vi "Waveform Example.vi"() -> ()   [LabVIEW 2016]
uses:
  controls/Microscope Settings.ctl
  controls/CameraState.ctl
  controls/ModeEnum.ctl
  <vilib>/DAQmx/write.llb/DAQmx Write (Digital 1D Wfm NChan NSamp).vi
  <vilib>/DAQmx/write.llb/DAQmx Write (Analog 1D Wfm NChan NSamp).vi
  <vilib>/Waveform/WDTOps.llb/WDT Number of Waveform Samples DBL.vi
  <vilib>/DAQmx/configure/timing.llb/DAQmx Timing (Sample Clock).vi
  <vilib>/Waveform/DWDTOps.llb/DWDT Uncompress Digital.vi
  <vilib>/DAQmx/miscellaneous.llb/DAQmx Fill In Error Info.vi
  <vilib>/Waveform/WDTOps.llb/WDT Waveform Duration DBL.vi
  <vilib>/DAQmx/create/channels.llb/DAQmx Create Channel (AO-Voltage-Basic).vi
  <vilib>/DAQmx/create/channels.llb/DAQmx Create Channel (DO-Digital Output).vi
  controls/PinOut.ctl
  controls/PinOut2.ctl
panel:
  out "Numeric 3":i32
  out "Numeric 2":i32
  in  "Tab Control":enum32{"Camera Settings", "Recording"}(tab)
  out "error IO":errorcluster
  out "Duration":string
  in  "Microscope Settings":T1={"Mode"=enum."XY", "Slit"={"Scanning Mode"=12.0, "Slit Width /%"=5.0}, "Colour"=[{"Laser"=enum."561", "Filter"=4}], "Exposure/ms"=40.0, "Piezo Position /um"=0.0, "ROI"={"X"={"Start /px"=0.0, "Step /px"=1.0, "Range /px"=2048.0}, "Y"={"Start /px"=0.0, "Step /px"=1.0, "Range /px"=2048.0}, "Z "={"Start /um"=0.0, "Step/um"=1.0, "Range /um"=100.0}, "T "={"Start /s"=0.0, "Step /s"=1.0, "Range /s"=100.0}}, "Samples per millisecond"=100.0, "Relax/ms"=10.0, "Readout Direction"=2.0, "Trigger Source"=2.0, "Camera Delay /ms"=11.0, "Under Scan /ms"=5.0, "Calibration Coordinates"={"Top Left"=[-4.418670520231216, -0.1592138728323702, 10.0], "Top Right"=[-9.501965317919073, -0.1592138728323702, 10.0], "Bottom Left"=[-4.4508670520231215, 0.0, 0.0], "Bottom Right"=[-9.53757225433526, 0.0, 0.0], "Waveforms"={"Analogue Out"=[], "Digital Out"=[]}}} {"Under Scan /ms" min=0.0 max=10.0 step=0.05; "ROI"."T"."Range /s" min=0.0 max=10.0 step=0.05 format="%<%H:%M:%S>t"; "ROI"."T"."Step /s" min=0.0 max=10.0 step=0.05 format="%<%M:%S%2u>t"; "ROI"."T"."Start /s" min=0.0 max=10.0 step=0.05 format="%<%M:%S%2u>t"; "ROI"."X"."Range /px" min=0.0 max=10.0 step=0.05; "ROI"."X"."Step /px" min=0.0 max=10.0 step=0.05; "ROI"."X"."Start /px" min=0.0 max=10.0 step=0.05; "ROI"."Y"."Range /px" min=0.0 max=10.0 step=0.05; "ROI"."Y"."Step /px" min=0.0 max=10.0 step=0.05; "ROI"."Y"."Start /px" min=0.0 max=10.0 step=0.05; "ROI"."Z"."Range /um" min=0.0 max=10.0 step=0.05; "ROI"."Z"."Step/um" min=0.0001 max=10.0 step=0.05; "ROI"."Z"."Start /um" min=0.0 max=10.0 step=0.05; "Colour"."Filter" items=["Empty"=1, ""=2, ""=3, "561"=4, ""=5, "488"=6]; "Camera Delay /ms" min=0.0 max=10.0 step=0.05; "Trigger Source" items=["Internal"=1.0, "External"=2.0]; "Readout Direction" items=["Forward"=1.0, "Backward"=2.0]; "Slit"."Scanning Mode" items=["Full Frame"=1.0, "Slit Scanning"=12.0]; "Piezo Position /um" min=0.0 max=10.0 step=0.05}
  out "Mixed Signal Graph 2":cluster{waveform(dbl)[], digitalwaveform[]}(graph)
  in  "stop":bool
  in  "Signals Debugger":bool
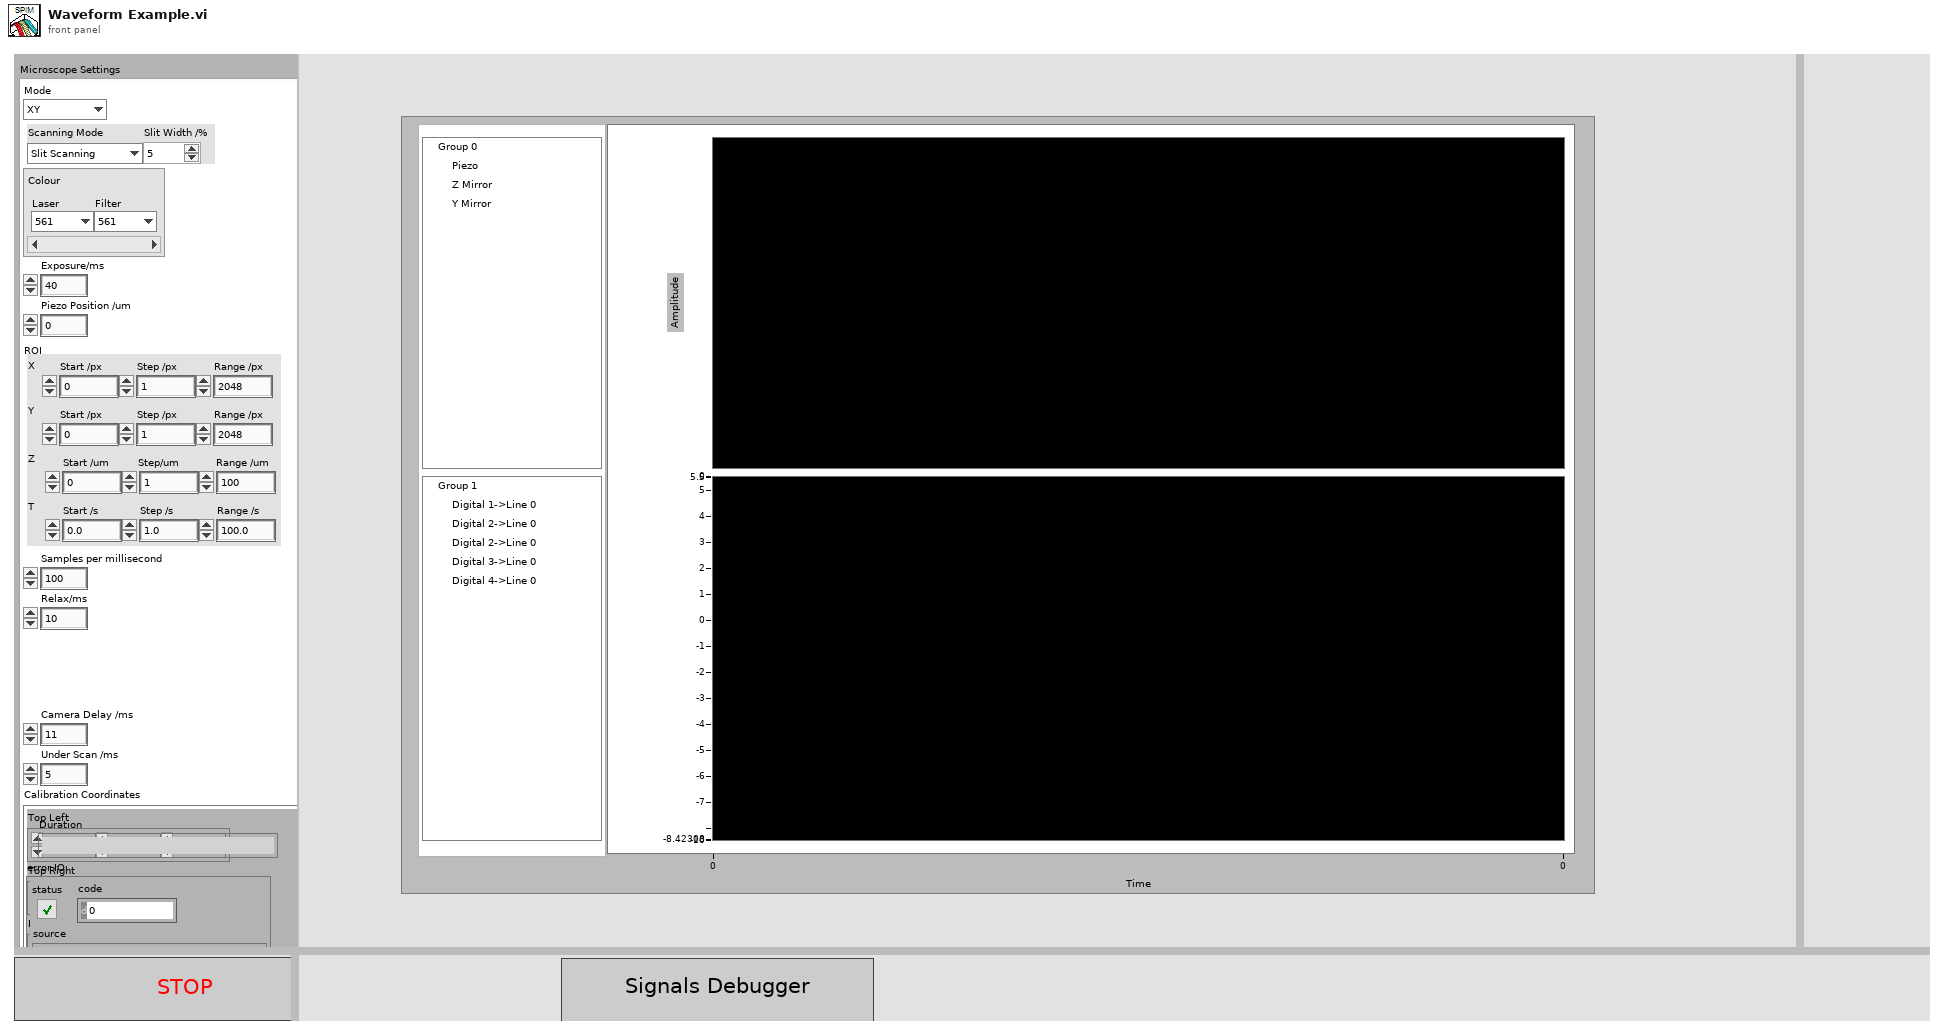
[diagram p1: front panel]
types:
  T1 = typedef "Microscope Settings.ctl" = cluster{"Mode":enum16{"Brightfield", "X", "XY", "XYZ", "XYZT", "XYZC", "Tweezers", "Virus"}, "Slit":cluster{"Scanning Mode":dbl, "Slit Width /%":dbl}, "Colour":cluster{"Laser":enum16{"Brightfield", "445", "488", "561", "647"}, "Filter":u16}[], "Exposure/ms":dbl, "Piezo Position /um":dbl, "ROI":cluster{"X":cluster{"Start /px":dbl, "Step /px":dbl, "Range /px":dbl}, "Y":cluster{"Start /px":dbl, "Step /px":dbl, "Range /px":dbl}, "Z ":cluster{"Start /um":dbl, "Step/um":dbl, "Range /um":dbl}, "T ":cluster{"Start /s":dbl, "Step /s":dbl, "Range /s":dbl}}, "Samples per millisecond":dbl, "Relax/ms":dbl, "Readout Direction":dbl, "Trigger Source":dbl, "Camera Delay /ms":dbl, "Under Scan /ms":dbl, "Calibration Coordinates":cluster{"Top Left":dbl[], "Top Right":dbl[], "Bottom Left":dbl[], "Bottom Right":dbl[], "Waveforms":cluster{"Analogue Out":waveform(dbl)[], "Digital Out":digitalwaveform[]}}}
  T2 = typedef "CameraState.ctl" = enum16{"init", "active", "deinit"}
  T3 = typedef "ModeEnum.ctl" = enum16{"Idle", "Init", "generateWaves", "runWaves", "runWavesCont", "endWavesCont", "stop"}
  T4 = enum16{"Stop", "Idle", "Update", "Run Waves", ""}
  T5 = typedef "PinOut.ctl" = string
  T6 = enum32{"Invalid", "Standard", "Closed", "Hidden", "Minimized", "Maximized"}
  T7 = cluster{"Analogue Out":waveform(dbl)[], "Digital Out":digitalwaveform[]}
  T8 = cluster{enum16{"Stop", "Idle", "Update", "Run Waves", ""}, "Microscope Settings":T1}
  T9 = typedef "PinOut2.ctl" = string
  T10 = enum16{"Brightfield", "X", "XY", "XYZ", "XYZT", "XYZC", "Tweezers", "Virus"}
  T11 = cluster{"Start /um":dbl, "Step/um":dbl, "Range /um":dbl}
  T12 = cluster{"Analogue Out out":waveform(dbl)[], "Digital Out out":digitalwaveform[]}
  T13 = cluster{"Start /s":dbl, "Step /s":dbl, "Range /s":dbl}
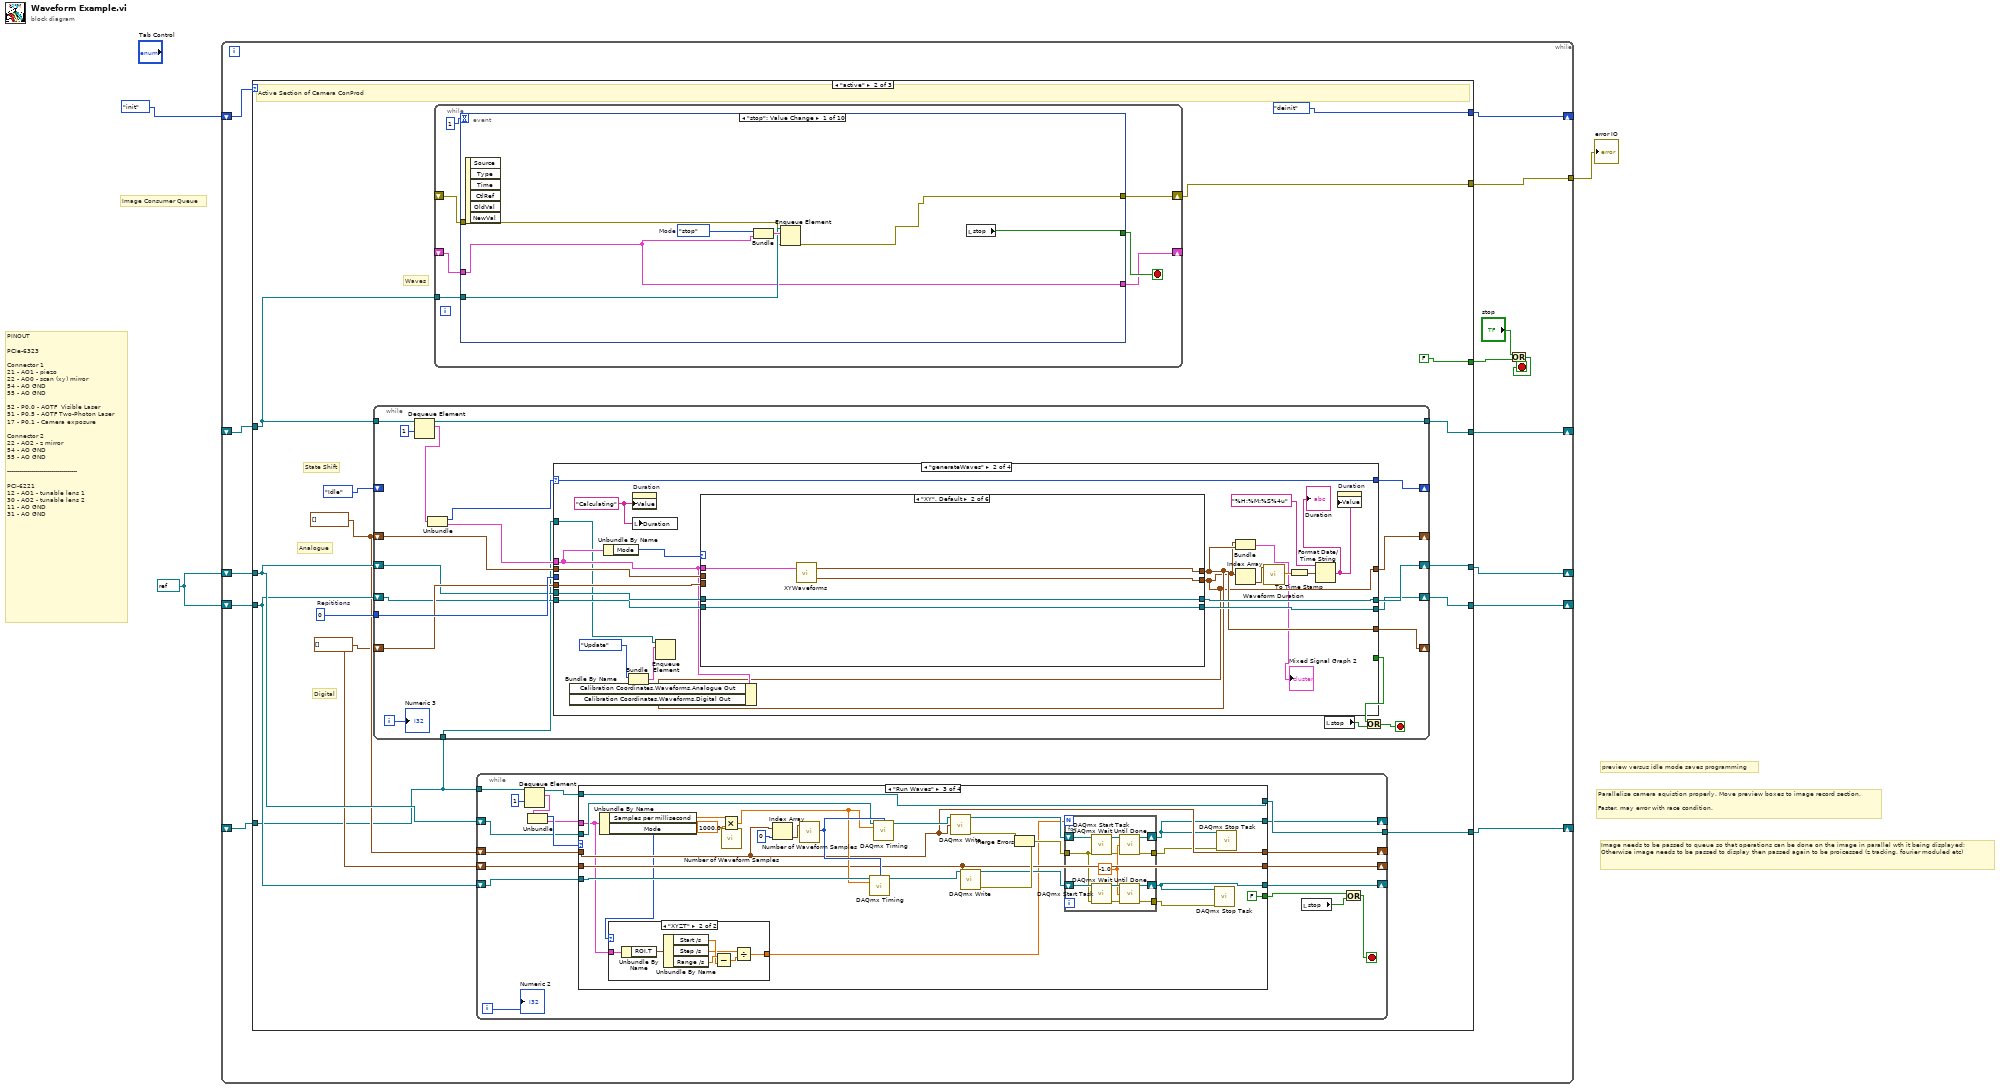
[diagram p0: block diagram]
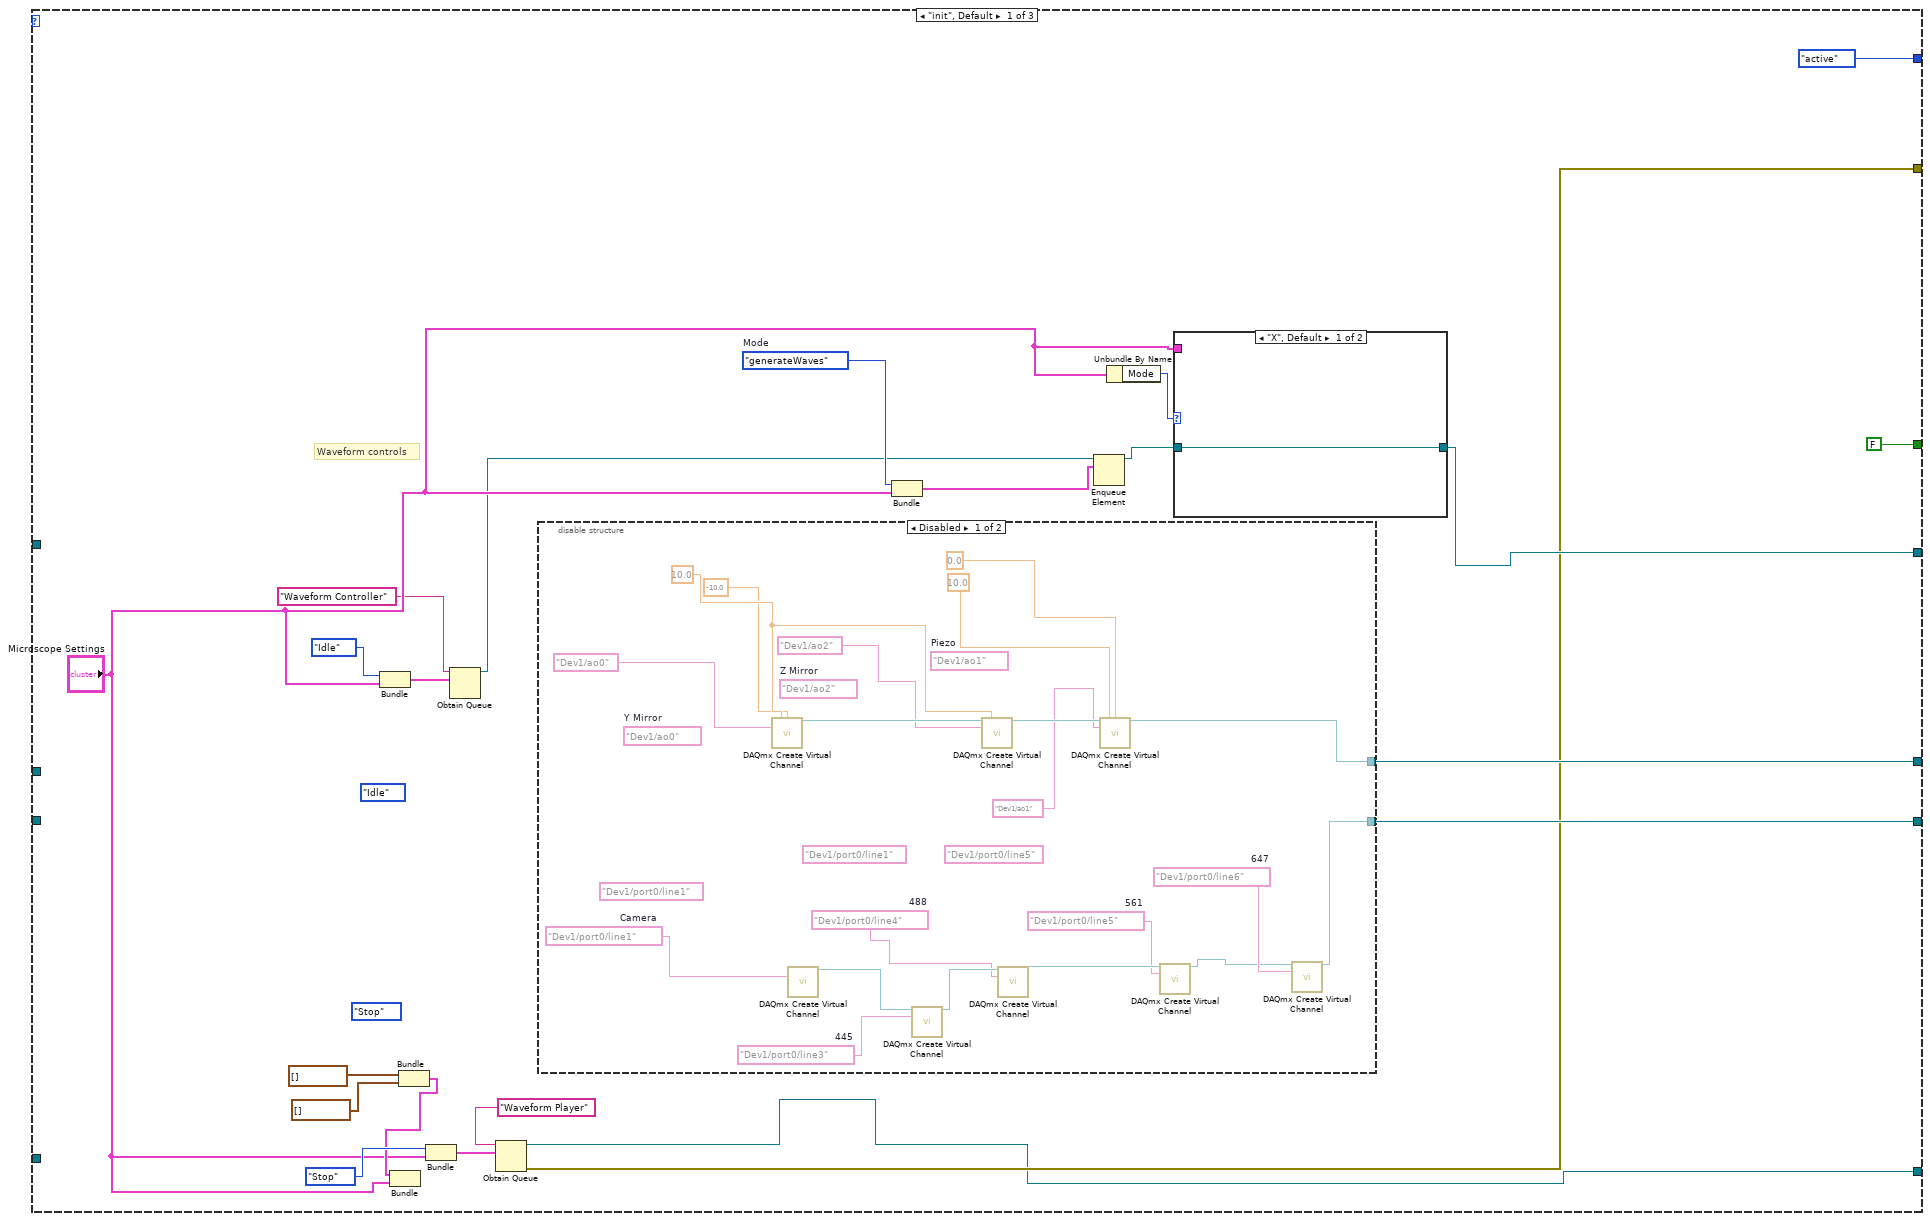
[diagram p2: hidden frame]
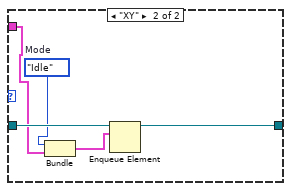
[diagram p4: hidden frame]
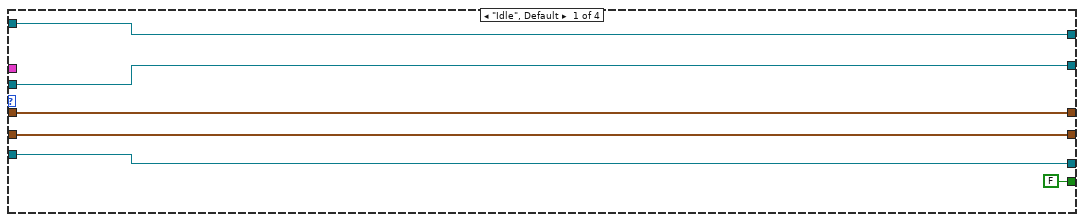
[diagram p5: hidden frame]
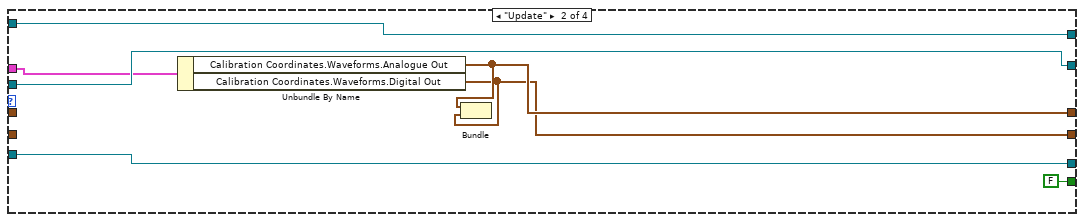
[diagram p6: hidden frame]
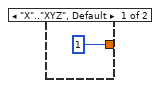
[diagram p7: hidden frame]
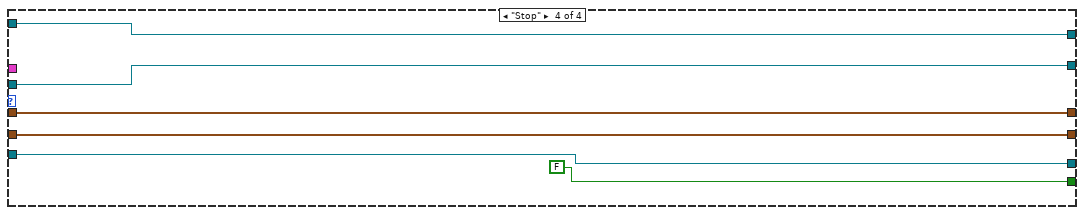
[diagram p8: hidden frame]
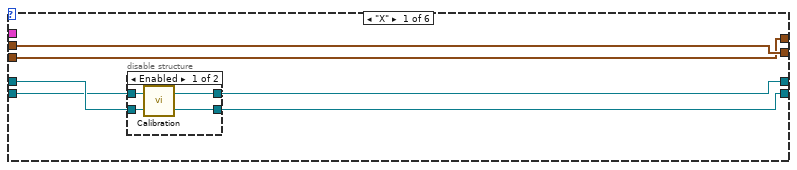
[diagram p10: hidden frame]
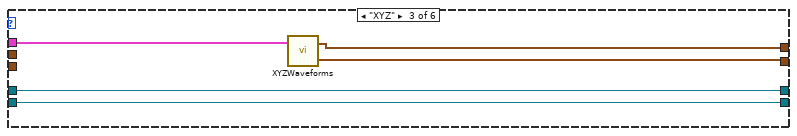
[diagram p12: hidden frame]
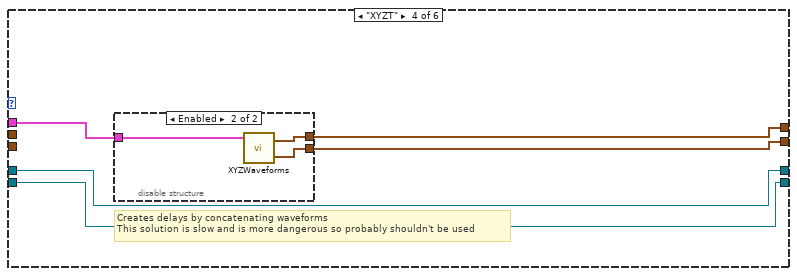
[diagram p13: hidden frame]
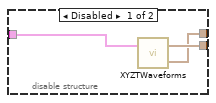
[diagram p14: hidden frame]
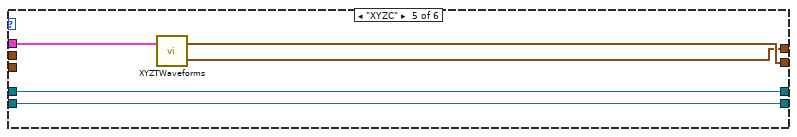
[diagram p15: hidden frame]
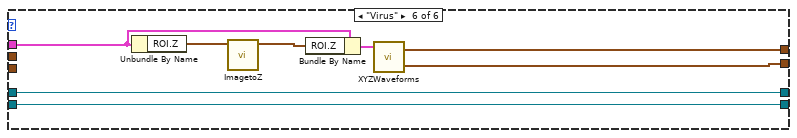
[diagram p16: hidden frame]
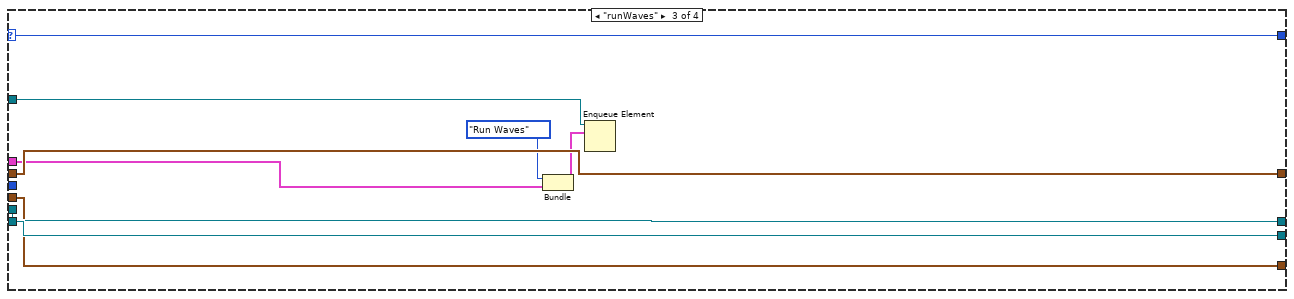
[diagram p17: hidden frame]
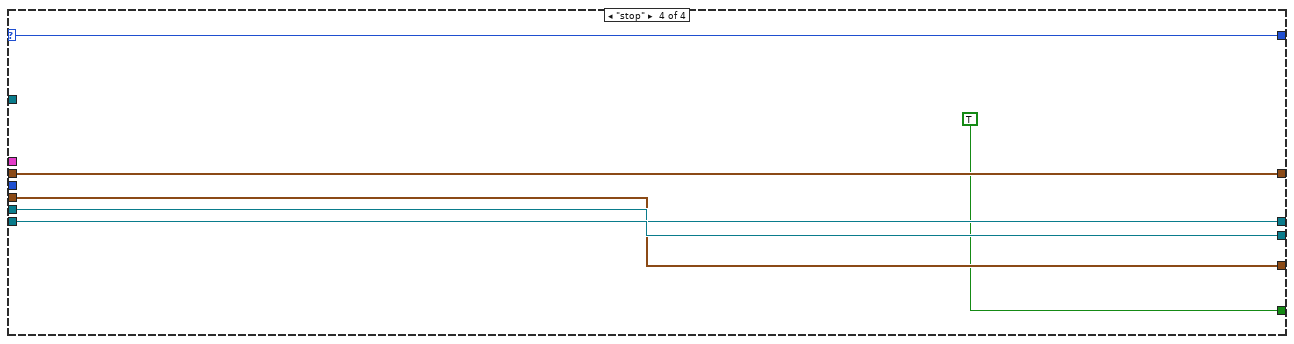
[diagram p18: hidden frame]
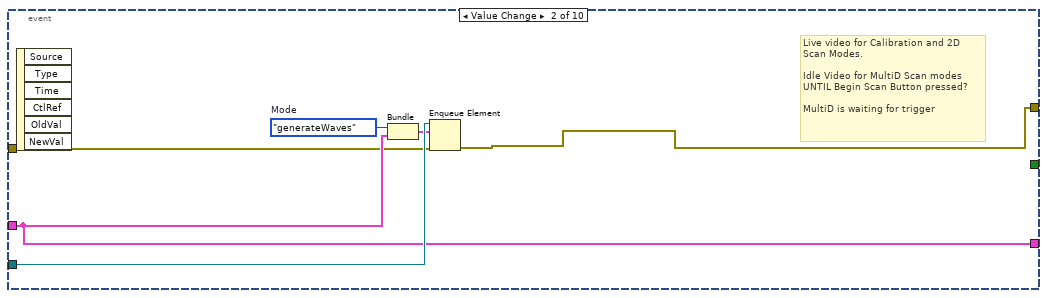
[diagram p19: hidden frame]
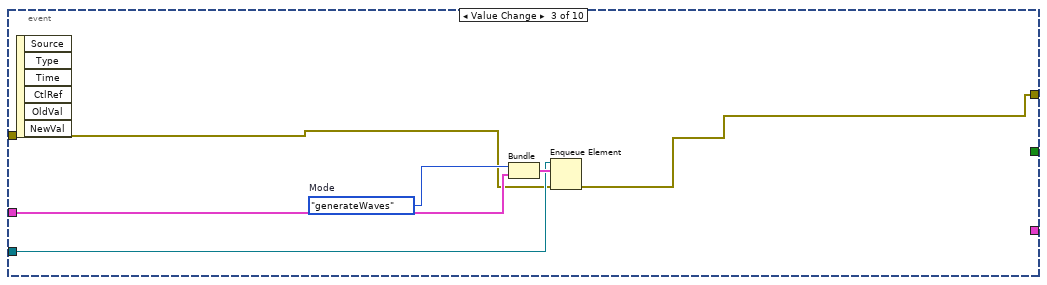
[diagram p20: hidden frame]
diagram:
  w2 = refnum<k21> refnum ("Mirror Z 2")
  # "PINOUT\n\nPCIe-6323\n\nConnector 1\n21 - AO1 - piezo\n22 - AO0 - scan (xy) mirror\n54 - AO GND\n55 - AO GND\n\n52 - P0.0 - AOTF  Visible Laser\n51 - P0.5 - AOTF Two-Photon Laser\n17 - P0.1 - Camera exposure\n\nConnector 2\n22 - AO2 - z mirror\n54 - AO GND\n55 - AO GND\n\n-----------------------------------\n\nPCI-6221\n12 - AO1 - tunable lens 1\n30 - AO2 - tunable lens 2\n11 - AO GND\n31 - AO GND"
  # "Image needs to be passed to queue so that operations can be done on the image in parallel wth it being displayed;\nOtherwise image needs to be passed to display then passed again to be proicessed (z tracking, fourier moduled etc)"
  # "preview versus idle mode saves programming"
  # "Parallelise camera aquistion properly. Move preview boxes to image record section.\n\nFaster. may error with race condition."
  # "Image Consumer Queue"
  n1 = while {
    shift-right: [w17] -> _
    shift-left: CameraState."init" -> [w5]
    shift-right: [w13] -> _
    shift-left: w2 -> [w12]
    shift-right: [w10] -> _
    shift-left: w2 -> [w11]
    shift-right: [w9] -> _
    shift-left: _ -> [w8]
    shift-right: [w7] -> _
    shift-left: _ -> [w6]
    tunnel: [w4] -> w1
    stop <- w15 stop-if-true
    n2 = case shown="\"active\"" w5 {
      selector: w5 -> [_ _ w341]
      tunnel: [CameraState."active" CameraState."deinit" w341] -> w17
      tunnel: [FALSE ("stop") FALSE ("stop") TRUE ("stop")] -> w14
      tunnel: w8 -> [_ w73 w344]
      tunnel: [w38 w76 w350] -> w13
      tunnel: w12 -> [_ w72 w350]
      tunnel: w11 -> [_ w71 w349]
      tunnel: [w37 w77 w349] -> w10
      tunnel: [w36 w75 w344] -> w9
      tunnel: [w18 w68 w343] -> w7
      tunnel: w6 -> [_ w67 w343]
      tunnel: [w19 w66 w342] -> w4
      frame "init", Default {
        (unwired) ModeEnum."Idle" ("Mode")
        w27 = ModeEnum."generateWaves"  # Mode
        (unwired) T4."Stop"
        # "Waveform controls"
        n3 = Bundle("Mode"=ModeEnum."Idle", "Microscope Settings"="Microscope Settings") -> (w25:cluster{"Mode":T3, "Microscope Settings":T1})  [unwired: 1 in]
        n4 = Bundle "Bundle"("Analogue Out"=waveform(dbl)[] [], "Digital Out"=digitalwaveform[] []) -> (w29:T7)  [unwired: 1 in]
        n5 = Bundle(w29, "Microscope Settings"="Microscope Settings") -> ()  [unwired: 1 in, 1 out]
        n6 = Bundle(T4."Stop", "Microscope Settings"="Microscope Settings") -> (w34:T8)  [unwired: 1 in]
        n7 = Obtain Queue(name (unnamed)="Waveform Controller", element data type=w25) -> (queue out=w24:refnum<queue>)  [unwired: 3 in, 2 out]
        n8 = Obtain Queue(name (unnamed)="Waveform Player", element data type=w34) -> (queue out=w18:refnum<queue>, error out=w19:errorcluster)  [unwired: 3 in, 1 out]
        n9 = disable-structure shown="Disabled" {
          disable-tunnel: [w59 _] -> w38
          disable-tunnel: [w58 _] -> w37
          frame Disabled {
            w41 = tag "Dev1/port0/line6"  # 647
            w43 = tag "Dev1/port0/line5"  # 561
            w48 = tag "Dev1/port0/line3"  # 445
            (unwired) T5 "Dev1/port0/line1" ("Combo Box")
            (unwired) T9 "Dev1/port0/line1" ("Combo Box")
            (unwired) T5 "Dev1/port0/line5" ("Combo Box")
            w45 = tag "Dev1/port0/line4"  # 488
            w42 = tag "Dev1/port0/line1"  # Camera
            (unwired) tag "Dev1/ao1"  # Piezo
            (unwired) tag "Dev1/ao2"  # Z Mirror
            (unwired) tag "Dev1/ao0"  # Y Mirror
            w57 = 10.0 ("maximum value")
            n10 = call-poly <vilib>:"DAQmx Create Virtual Channel.vi"("maximum value"=w57, "minimum value"=-10.0, "physical channels"=T5 "Dev1/ao0" ("Combo Box")) -> ("task out"=w53:refnum<k21>)  [unwired: 11 in, 1 out]
            n11 = call-poly <vilib>:"DAQmx Create Virtual Channel.vi"("lines"=w42) -> ("task out"=w47:refnum<k21>)  [unwired: 13 in, 1 out]
            n12 = call-poly <vilib>:"DAQmx Create Virtual Channel.vi"("task in"=w47, "lines"=w48) -> ("task out"=w46:refnum<k21>)  [unwired: 12 in, 1 out]
            n13 = call-poly <vilib>:"DAQmx Create Virtual Channel.vi"("task in"=w53, "maximum value"=w57, "physical channels"=T5 "Dev1/ao2" ("Combo Box")) -> ("task out"=w52:refnum<k21>)  [unwired: 11 in, 1 out]
            n14 = call-poly <vilib>:"DAQmx Create Virtual Channel.vi"("task in"=w46, "lines"=w45) -> ("task out"=w44:refnum<k21>)  [unwired: 12 in, 1 out]
            n15 = call-poly <vilib>:"DAQmx Create Virtual Channel.vi"("task in"=w52, "maximum value"=10.0 ("minimum value"), "minimum value"=0.0 ("maximum value"), "physical channels"=T5 "Dev1/ao1" ("Combo Box")) -> ("task out"=w59:refnum<k21>)  [unwired: 10 in, 1 out]
            n16 = call-poly <vilib>:"DAQmx Create Virtual Channel.vi"("task in"=w44, "lines"=w43) -> ("task out"=w40:refnum<k21>)  [unwired: 12 in, 1 out]
            n17 = call-poly <vilib>:"DAQmx Create Virtual Channel.vi"("task in"=w40, "lines"=w41) -> ("task out"=w58:refnum<k21>)  [unwired: 12 in, 1 out]
          }
          frame Enabled {
          }
        }
        n18 = Bundle("Mode"=w27, "Microscope Settings"="Microscope Settings") -> (w21:cluster{"Mode":T3, "Microscope Settings":T1})  [unwired: 1 in]
        n19 = Enqueue Element(queue=w24, element=w21) -> (queue out=w22:refnum<queue>)  [unwired: 2 in, 2 out]
        n20 = Unbundle By Name("Microscope Settings") -> ("Mode"=w20:T10)
        n21 = case shown="\"X\", Default" w20 {
          tunnel: w22 -> [w60 w65]
          tunnel: "Microscope Settings" -> [_ w63]
          tunnel: [w60 w61] -> w36
          frame "X", Default {
          }
          frame "XY" {
            w62 = ModeEnum."Idle"  # Mode
            n22 = Bundle("Mode"=w62, "Microscope Settings"=w63) -> (w64:cluster{"Mode":T3, "Microscope Settings":T1})  [unwired: 1 in]
            n23 = Enqueue Element(queue=w65, element=w64) -> (queue out=w61:refnum<queue>)  [unwired: 2 in, 2 out]
          }
        }
      }
      frame "active" {
        w69 = digitalwaveform[] [] ("Digital Out")
        w70 = waveform(dbl)[] [] ("Analogue Out")
        w78 = 0  # Repititions
        # "State Shift"
        # "Waves"
        # "Digital"
        # "Analogue"
        # "Active Section of Camera ConProd"
        n24 = while {
          tunnel: w73 -> [w185]
          shift-right: [w184] -> _
          shift-left: w70 -> [w183]
          tunnel: w78 -> [w182]
          shift-right: [w178] -> w76
          shift-left: w72 -> [w177]
          shift-right: [w181] -> _
          shift-left: w69 -> [w180]
          shift-right: [w176] -> w77
          shift-left: w71 -> [w175]
          tunnel: [w174] -> w75
          shift-right: [w170] -> _
          shift-left: ModeEnum."Idle" ("Mode") -> [_]
          tunnel: w67 -> [w166]
          i -> [w165]
          stop <- w171 stop-if-true
          n25 = Dequeue Element(queue=w185, timeout in ms (-1)=1) -> (queue out=w174:refnum<queue>, element=w169:cluster{"Mode":T3, "Microscope Settings":T1})  [unwired: 1 in, 2 out]
          n26 = Unbundle(w169) -> ("Mode"=w168:T3, "Microscope Settings"=w167:T1)
          n27 = case shown="\"generateWaves\"" w168 {
            selector: w168 -> [w186 w199 w265 w268]
            tunnel: [_ _ _ TRUE] -> w173
            tunnel: w167 -> [_ w197 w260 _]
            tunnel: [w190 w192 w263 w273] -> w184
            tunnel: w183 -> [w190 w210 w263 w273]
            tunnel: w182 -> [_ _ _ _]
            tunnel: [w187 w200 w267 w272] -> w176
            tunnel: [w188 w202 w266 w271] -> w178
            tunnel: w177 -> [w188 w203 w266 w271]
            tunnel: [w189 w193 w262 w270] -> w181
            tunnel: w180 -> [w189 w212 w262 w270]
            tunnel: w175 -> [w187 w201 w267 w272]
            tunnel: [w186 w199 w265 w268] -> w170
            tunnel: w166 -> [_ w194 w264 _]
            frame "Idle", Default {
            }
            frame "generateWaves" {
              w205 = "Calculating" ("date/time string")
              n28 = Unbundle By Name(w197) -> ("Mode"=w211:T10)
              n29 = property on="Duration" class="Str"("Value"=w205) -> ()  [unwired: 2 in, 2 out]
              n30 = local write "Duration"(w205) -> ()
              n31 = case shown="\"XY\", Default" w211 {
                tunnel: [w218 w228 w231 w239 w249 w255] -> w192
                tunnel: w197 -> [_ w229 w232 w237 w250 w254]
                tunnel: [w217 w227 w230 w238 w248 w256] -> w193
                tunnel: w212 -> [w217 _ _ _ _ _]
                tunnel: w210 -> [w218 _ _ _ _ _]
                tunnel: w203 -> [w216 w226 w234 w236 w247 w258]
                tunnel: w201 -> [w215 w225 w233 w235 w246 w257]
                tunnel: [w214 w226 w234 w236 w247 w258] -> w202
                tunnel: [w213 w225 w233 w235 w246 w257] -> w200
                frame "X" {
                  n32 = disable-structure shown="Enabled" {
                    disable-tunnel: w216 -> [w222 w223]
                    disable-tunnel: w215 -> [w221 w224]
                    disable-tunnel: [w220 w224] -> w214
                    disable-tunnel: [w219 w223] -> w213
                    frame Enabled {
                      n33 = call "Calibration.vi"("Analogue In"=w222, "Digital In"=w221) -> ("Analogue In Out"=w219:refnum<k21>, "Digital Out"=w220:refnum<k21>)
                    }
                    frame Disabled {
                    }
                  }
                }
                frame "XY", Default {
                  n34 = call "XYWaveforms.vi"("Microscope Settings"=w229) -> ("Analogue Out"=w228:waveform(dbl)[], "Digital Out"=w227:digitalwaveform[])  [unwired: 1 out]
                }
                frame "XYZ" {
                  n35 = call "XYZWaveforms.vi"("Microscope Settings"=w232) -> ("Analogue Out out"=w231:waveform(dbl)[], "Digital Out out"=w230:digitalwaveform[])  [unwired: 2 in]
                }
                frame "XYZT" {
                  # "Creates delays by concatenating waveforms\nThis solution is slow and is more dangerous so probably shouldn't be used"
                  n36 = disable-structure shown="Enabled" {
                    disable-tunnel: [w242 w243] -> w239
                    disable-tunnel: [w241 w244] -> w238
                    disable-tunnel: w237 -> [w240 w245]
                    frame Disabled {
                      n37 = call "XYZTWaveforms.vi"("Microscope Settings"=w240) -> ("Digital Out"=w241:digitalwaveform[], "Analogue Out"=w242:waveform(dbl)[])  [unwired: 1 in]
                    }
                    frame Enabled {
                      n38 = call "XYZWaveforms.vi"("Microscope Settings"=w245) -> ("Analogue Out out"=w243:waveform(dbl)[], "Digital Out out"=w244:digitalwaveform[])  [unwired: 2 in]
                    }
                  }
                }
                frame "XYZC" {
                  n39 = call "XYZTWaveforms.vi"("Microscope Settings"=w250) -> ("Digital Out"=w248:digitalwaveform[], "Analogue Out"=w249:waveform(dbl)[])  [unwired: 1 in]
                }
                frame "Virus" {
                  n40 = Unbundle By Name(w254) -> ("ROI.Z"=w252:T11)
                  n41 = call "ImagetoZ.vi"("Z"=w252) -> ("ROI.Z"=w251:T11)  [unwired: 10 in]
                  n42 = Bundle By Name(cluster=w254, "ROI.Z"=w251) -> (w253:T1)
                  n43 = call "XYZWaveforms.vi"("Microscope Settings"=w253) -> ("Analogue Out out"=w255:waveform(dbl)[], "Digital Out out"=w256:digitalwaveform[])  [unwired: 2 in]
                }
              }
              n44 = Bundle By Name(cluster=w197, "Calibration Coordinates.Waveforms.Analogue Out"=w192, "Calibration Coordinates.Waveforms.Digital Out"=w193) -> (w196:T1)
              n45 = Bundle(T4."Update", "Microscope Settings"=w196) -> (w195:T8)  [unwired: 1 in]
              n46 = Enqueue Element(queue=w194, element=w195) -> ()  [unwired: 2 in, 3 out]
              n47 = Bundle("Analogue Out out"=w192, "Digital Out out"=w193) -> (→"Mixed Signal Graph 2":T12)  [unwired: 1 in]
              n48 = Index Array(array=w192) -> (element=w209:waveform(dbl))  [unwired: 1 in]
              n49 = call-poly <vilib>:"Waveform Duration.vi"("waveform in"=w209) -> ("duration"=w207:dbl)  [unwired: 8 in, 2 out]
              n50 = To Time Stamp(1:w207) -> (0:w208:timestamp)
              n51 = Format Date/Time String(time format string (%c)="%H:%M:%S%4u", seconds (now)=w208) -> (date/time string=w204:string)  [unwired: 1 in]
              "Duration" <- w204
              n52 = property on="Duration" class="Str"("Value"=w204) -> ()  [unwired: 2 in, 2 out]
            }
            frame "runWaves" {
              n53 = Bundle(T4."Run Waves", "Microscope Settings"=w260) -> (w259:T8)  [unwired: 1 in]
              n54 = Enqueue Element(queue=w264, element=w259) -> ()  [unwired: 2 in, 3 out]
            }
            frame "stop" {
            }
          }
          n55 = local read "stop"() -> (w172:bool)
          n56 = Or(x=w173, y=w172) -> (x .or. y?=w171:bool)
          "Numeric 3" <- w165
        }
        n57 = while {
          shift-right: [w279] -> _
          shift-left: _ -> [w278]
          tunnel: w73 -> [w276]
          shift-right: [w275] -> w66
          shift-left: _ -> [w274]
          stop <- w280 stop-if-true
          n58 = event shown="[0] \"stop\": Value Change" {
            selector: _ -> [_ _ _ _ _ _ _ _ _ _]
            dyn-events: _ -> [_ _ _ _ _ _ _ _ _ _]
            timeout: 1 -> [_ _ _ _ _ _ _ _ _ _]
            tunnel: [w287 _ _ _ _ _ _ _ _ _] -> w280
            tunnel: [w283 w290 _ _ _ _ _ _ _ w340] -> w279
            tunnel: w278 -> [w283 w290 w297 w302 w309 w316 w321 w327 _ _]
            tunnel: w276 -> [w284 w293 w298 w303 w308 w312 w322 w326 _ _]
            tunnel: [w281 w288 w294 w300 w306 w314 w319 w324 w331 w339] -> w275
            tunnel: w274 -> [w282 w289 w295 w301 w307 w315 w318 w325 w330 w339]
            event "stop": Value Change {
              w286 = ModeEnum."stop"  # Mode
              n59 = event-data() -> ()  [unwired: 1 in, 6 out]
              n60 = Bundle("Mode"=w286, "Value"=w283) -> (w285:cluster{"Mode":T3, "Value":T1})  [unwired: 1 in]
              n61 = Enqueue Element(queue=w284, element=w285, error in (no error)=w282) -> (error out=w281:errorcluster)  [unwired: 1 in, 2 out]
              n62 = local read "stop"() -> (w287:bool)
            }
            event Value Change {
              w292 = ModeEnum."generateWaves"  # Mode
              # "Live video for Calibration and 2D\nScan Modes.\n\nIdle Video for MultiD Scan modes\nUNTIL Begin Scan Button pressed?\n\nMultiD is waiting for trigger"
              n63 = event-data() -> ()  [unwired: 1 in, 6 out]
              n64 = Bundle("Mode"=w292, "Value"=w290) -> (w291:cluster{"Mode":T3, "Value":T1})  [unwired: 1 in]
              n65 = Enqueue Element(queue=w293, element=w291, error in (no error)=w289) -> (error out=w288:errorcluster)  [unwired: 1 in, 2 out]
            }
            event Value Change {
              w296 = ModeEnum."generateWaves"  # Mode
              n66 = event-data() -> ()  [unwired: 1 in, 6 out]
              n67 = Bundle("Mode"=w296, "Value"=w297) -> (w299:cluster{"Mode":T3, "Value":T1})  [unwired: 1 in]
              n68 = Enqueue Element(queue=w298, element=w299, error in (no error)=w295) -> (error out=w294:errorcluster)  [unwired: 1 in, 2 out]
            }
            event Value Change {
              w304 = ModeEnum."generateWaves"  # Mode
              n69 = event-data() -> ()  [unwired: 1 in, 6 out]
              n70 = Bundle("Mode"=w304, "Value"=w302) -> (w305:cluster{"Mode":T3, "Value":T1})  [unwired: 1 in]
              n71 = Enqueue Element(queue=w303, element=w305, error in (no error)=w301) -> (error out=w300:errorcluster)  [unwired: 1 in, 2 out]
            }
            event Value Change {
              w311 = ModeEnum."generateWaves"  # Mode
              n72 = event-data() -> ()  [unwired: 1 in, 6 out]
              n73 = Bundle("Mode"=w311, "Value"=w309) -> (w310:cluster{"Mode":T3, "Value":T1})  [unwired: 1 in]
              n74 = Enqueue Element(queue=w308, element=w310, error in (no error)=w307) -> (error out=w306:errorcluster)  [unwired: 1 in, 2 out]
            }
            event Value Change {
              w317 = ModeEnum."generateWaves"  # Mode
              n75 = event-data() -> ()  [unwired: 1 in, 6 out]
              n76 = Bundle("Mode"=w317, "Value"=w316) -> (w313:cluster{"Mode":T3, "Value":T1})  [unwired: 1 in]
              n77 = Enqueue Element(queue=w312, element=w313, error in (no error)=w315) -> (error out=w314:errorcluster)  [unwired: 1 in, 2 out]
            }
            event Value Change {
              w323 = ModeEnum."generateWaves"  # Mode
              n78 = event-data() -> ()  [unwired: 1 in, 6 out]
              n79 = Bundle("Mode"=w323, "Value"=w321) -> (w320:cluster{"Mode":T3, "Value":T1})  [unwired: 1 in]
              n80 = Enqueue Element(queue=w322, element=w320, error in (no error)=w318) -> (error out=w319:errorcluster)  [unwired: 1 in, 2 out]
            }
            event Value Change {
              w329 = ModeEnum."generateWaves"  # Mode
              n81 = event-data() -> ()  [unwired: 1 in, 6 out]
              n82 = Bundle("Mode"=w329, "Value"=w327) -> (w328:cluster{"Mode":T3, "Value":T1})  [unwired: 1 in]
              n83 = Enqueue Element(queue=w326, element=w328, error in (no error)=w325) -> (error out=w324:errorcluster)  [unwired: 1 in, 2 out]
            }
            event "Signals Debugger": Value Change {
              n84 = event-data() -> ()  [unwired: 1 in, 6 out]
              n85 = case shown="True" "Signals Debugger" {
                tunnel: [w333 w335] -> w331
                tunnel: w330 -> [w333 w334]
                frame False {
                }
                frame True {
                  n86 = vi-ref "Graph.vi"() -> (w336:refnum<vi>)
                  n87 = invoke class="VI" method="FP.Open"(reference=w336, error in=w334, "Activate"=TRUE ("Front Panel Window:Open"), "State"=T6."Standard") -> (error out=w335:errorcluster)  [unwired: 1 in, 4 out]
                }
              }
            }
            event Timeout {
              n88 = event-data() -> ()  [unwired: 1 in, 3 out]
              n89 = property on="Microscope Settings" class="Clust (strict)"() -> ("Value"=w340:T1)  [unwired: 2 in, 2 out]
            }
          }
        }
        n90 = while {
          tunnel: [w98] -> w68
          tunnel: w67 -> [w97]
          shift-right: [w93] -> _
          shift-left: w70 -> [w91]
          shift-right: [w92] -> _
          shift-left: w69 -> [w90]
          shift-right: [w83] -> _
          shift-left: w71 -> [w85]
          shift-right: [w84] -> _
          shift-left: w72 -> [w86]
          i -> [w82]
          stop <- w88 stop-if-true
          n91 = Dequeue Element(queue=w97, timeout in ms (-1)=1) -> (queue out=w96:refnum<queue>, element=w95:T8)  [unwired: 1 in, 2 out]
          n92 = Unbundle(w95) -> (w94:T4, "Microscope Settings"=w89:T1)
          n93 = case shown="\"Run Waves\"" w94 {
            tunnel: [w105 w112 w138 w162] -> w98
            tunnel: w96 -> [w105 w112 w138 w162]
            tunnel: w89 -> [_ w108 w120 _]
            tunnel: [w104 w107 w121 w164] -> w93
            tunnel: [w103 w106 w122 w163] -> w92
            tunnel: w91 -> [w104 _ w121 w164]
            tunnel: w90 -> [w103 _ w122 w163]
            tunnel: [FALSE FALSE FALSE FALSE] -> w87
            tunnel: w86 -> [w102 w111 w132 w160]
            tunnel: w85 -> [w101 w110 w131 w159]
            tunnel: [w102 w111 w117 w160] -> w84
            tunnel: [w101 w110 w114 w159] -> w83
            frame "Idle", Default {
            }
            frame "Update" {
              n94 = Unbundle By Name(w108) -> ("Calibration Coordinates.Waveforms.Analogue Out"=w107:waveform(dbl)[], "Calibration Coordinates.Waveforms.Digital Out"=w106:digitalwaveform[])
              n95 = Bundle("Analogue Out"=w107, "Digital Out"=w106) -> ()  [unwired: 1 in, 1 out]
            }
            frame "Run Waves" {
              n96 = Unbundle By Name(w120) -> ("Samples per millisecond"=w136:dbl, "Mode"=w119:T10)
              n97 = case shown="\"XYZT\"" w119 {
                tunnel: [1 w140] -> w118
                tunnel: w120 -> [_ w146]
                frame "X".."XYZ", Default {
                }
                frame "XYZT" {
                  n98 = Unbundle By Name(w146) -> ("ROI.T"=w145:T13)
                  n99 = Unbundle By Name(w145) -> ("Start /s"=w143:dbl, "Step /s"=w141:dbl, "Range /s"=w144:dbl)
                  n100 = Subtract(x=w144, y=w143) -> (x-y=w142:dbl)
                  n101 = Divide(x=w141, y=w142) -> (x/y=w140:dbl)
                }
              }
              n102 = Multiply(x=w136, y=1000.0) -> (x*y=w130:dbl)
              n103 = call-poly <vilib>:"Number of Waveform Samples.vi"() -> ()  [unwired: 9 in, 3 out]
              n104 = Index Array(array=w121, index=0) -> (element=w134:waveform(dbl))
              n105 = call-poly <vilib>:"Number of Waveform Samples.vi"("waveform in"=w134) -> ("number of samples"=w133:i32)  [unwired: 8 in, 2 out]
              n106 = call-poly <vilib>:"DAQmx Timing.vi"("task/channels in"=w131, "samples per channel"=w133, "rate"=w130) -> ("task out"=w128:refnum<k21>)  [unwired: 11 in, 1 out]
              n107 = call-poly <vilib>:"DAQmx Timing.vi"("task/channels in"=w132, "samples per channel"=w133, "rate"=w130) -> ("task out"=w129:refnum<k21>)  [unwired: 11 in, 1 out]
              n108 = call-poly <vilib>:"DAQmx Write.vi"("task/channels in"=w129, "data"=w121) -> ("task out"=w125:refnum<k21>, "error out"=w127:errorcluster)  [unwired: 11 in, 1 out]
              n109 = call-poly <vilib>:"DAQmx Write.vi"("task/channels in"=w128, "data"=w122) -> ("task out"=w124:refnum<k21>, "error out"=w126:errorcluster)  [unwired: 11 in, 1 out]
              n110 = Merge Errors(w127, w126) -> (w123:errorcluster)
              n111 = for {
                N: w118 -> [_]
                tunnel: w123 -> [w152]
                shift-right: [w155] -> w117
                shift-left: w125 -> [w158]
                shift-right: [w153] -> w114
                shift-left: w124 -> [w157]
                tunnel: [w148] -> w115
                tunnel: [w147] -> w116
                w151 = -1.0 ("timeout (sec)")
                n112 = call <vilib>:"DAQmx Start Task.vi"("task/channels in"=w158, "error in"=w152) -> ("task out"=w156:refnum<k21>, "error out"=w150:errorcluster)  [unwired: 12 in]
                n113 = call <vilib>:"DAQmx Start Task.vi"("task/channels in"=w157, "error in"=w152) -> ("task out"=w154:refnum<k21>, "error out"=w149:errorcluster)  [unwired: 12 in]
                n114 = call <vilib>:"DAQmx Wait Until Done.vi"("task/channels in"=w156, "timeout (sec)"=w151, "error in"=w150) -> ("task out"=w155:refnum<k21>, "error out"=w147:errorcluster)  [unwired: 11 in]
                n115 = call <vilib>:"DAQmx Wait Until Done.vi"("task/channels in"=w154, "timeout (sec)"=w151, "error in"=w149) -> ("task out"=w153:refnum<k21>, "error out"=w148:errorcluster)  [unwired: 11 in]
              }
              n116 = call <vilib>:"DAQmx Stop Task.vi"("task/channels in"=w114, "error in"=w115) -> ()  [unwired: 12 in, 2 out]
              n117 = call <vilib>:"DAQmx Stop Task.vi"("task/channels in"=w117, "error in"=w116) -> ()  [unwired: 12 in, 2 out]
            }
            frame "Stop" {
            }
          }
          n118 = local read "stop"() -> (w99:bool)
          n119 = Or(x=w87, y=w99) -> (x .or. y?=w88:bool)
          "Numeric 2" <- w82
        }
      }
      frame "deinit" {
        n120 = disable-structure shown="Enabled" {
          disable-tunnel: w350 -> [w356 _]
          disable-tunnel: w349 -> [w354 _]
          disable-tunnel: [w353 _] -> w347
          disable-tunnel: [w352 _] -> w346
          frame Disabled {
            n121 = call <vilib>:"DAQmx Stop Task.vi"("task/channels in"=w354) -> ("task out"=w355:refnum<k21>)  [unwired: 13 in, 1 out]
            n122 = call <vilib>:"DAQmx Stop Task.vi"("task/channels in"=w356) -> ("task out"=w357:refnum<k21>)  [unwired: 13 in, 1 out]
            n123 = call <vilib>:"DAQmx Clear Task.vi"("task in"=w355) -> ("error out"=w352:errorcluster)  [unwired: 14 in]
            n124 = call <vilib>:"DAQmx Clear Task.vi"("task in"=w357) -> ("error out"=w353:errorcluster)  [unwired: 14 in]
          }
          frame Enabled {
          }
        }
        n125 = Flush Queue(queue=w344) -> (queue out=w345:refnum<queue>)  [unwired: 1 in, 2 out]
        n126 = Release Queue(queue=w345) -> (error out=w348:errorcluster)  [unwired: 2 in, 2 out]
        n127 = Merge Errors(w348, w347, w346) -> (w342:errorcluster)
      }
    }
    n128 = Or(x="stop", y=w14) -> (x .or. y?=w15:bool)
  }
  "error IO" <- w1
